vi "Start.vi"(8 "error in":errorcluster, 11 "Tx Execution Unit Implementation in":refnum<class "Tx Generic Execution Unit.lvclass">) -> (0 "error out":errorcluster, 3 "Tx Execution Unit Implementation out":refnum<class "Tx Generic Execution Unit.lvclass">)   [LabVIEW 2020, in "AIM ARINC 664 Engine.lvlib" / "Implementation.lvlib" / "Tx Generic Execution Unit.lvclass"]
uses:
  Tx Generic Execution Unit.lvclass
  <instrlib>/AIM GmbH/_AIM 664/AIM664LV.lvlib
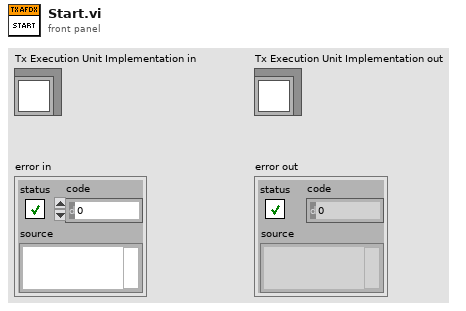
[diagram p1: front panel]
types:
  T1 = cluster{"StartMode":i32, "Count":u32, "Sign":i32, "Day":u32, "Hour":u32, "Min":u32, "Second":u32, "MilliSec":u32, "MicroSec":u32, "ExtendedStopMode":i32, "TransmitTime":u32}
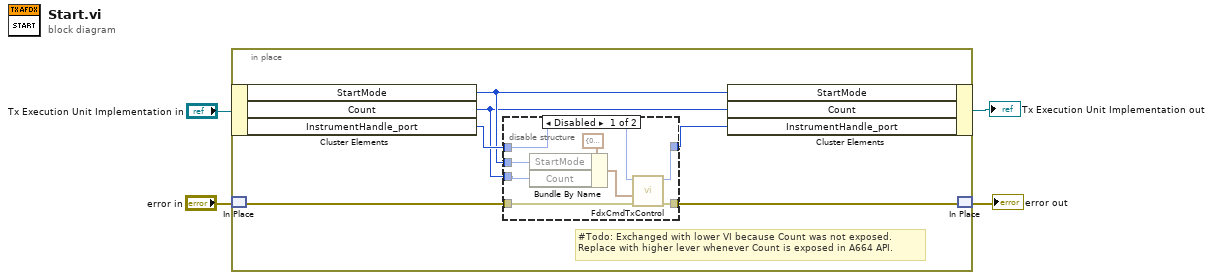
[diagram p0: block diagram]
diagram:
  n1 = in-place {
    # "#Todo: Exchanged with lower VI because Count was not exposed.\nReplace with higher lever whenever Count is exposed in A664 API."
    n2 = in-place-cluster #1("Tx Execution Unit Implementation in") -> ("StartMode"=w6:u32, "Count"=w5:u32, "InstrumentHandle_port"=w10:u32)
    n3 = in-place-match #2("error in") -> (w8:errorcluster)
    n4 = disable-structure shown="Disabled" {
      disable-tunnel: w10 -> [w18 w19]
      disable-tunnel: [w17 w19] -> w9
      disable-tunnel: w8 -> [w16 w20]
      disable-tunnel: [w15 w20] -> w7
      disable-tunnel: w6 -> [w12 _]
      disable-tunnel: w5 -> [w11 _]
      frame Disabled {
        n5 = Bundle By Name(cluster=T1 {"StartMode"=0, "Count"=0, "Sign"=0, "Day"=0, "Hour"=0, "Min"=0, "Second"=0, "MilliSec"=0, "MicroSec"=0, "ExtendedStopMode"=0, "TransmitTime"=0} ("TxControl"), "StartMode"=w12, "Count"=w11) -> (w13:T1)
        n6 = call <instrlib>:"FdxCmdTxControl.vi"("error in"=w16, "TxControl"=w13, "InstrumentHandle_port in"=w18) -> ("error out"=w15:errorcluster, "InstrumentHandle_port out"=w17:u32)  [unwired: 7 in]
      }
      frame Enabled {
      }
    }
    n7 = in-place-cluster #1("StartMode"=w6, "Count"=w5, "InstrumentHandle_port"=w9) -> (→"Tx Execution Unit Implementation out":refnum<class "Tx Generic Execution Unit.lvclass">)
    n8 = in-place-match #2(w7) -> (→"error out":errorcluster)
  }
